vi "PRIME FITS Add Observer Info.vi"(8 "Error In":errorcluster, 10 "Observation":T2={"Priority"=0, "ID"="", "Observer"="", "Obj Name"="", "Obj Type"="", "RA and DEC String"={"RA"="HH:MM:SS.nnn", "DEC"="DEG:arcmin:arcsec.nn"}, "Filter Wheel 1"="", "Filter Wheel 2"="", "Integration Time"=0.0, "Observation Status"=enum."Error", "Offsets"={"RA"=0.0, "DEC"=0.0, "ROT"=0.0}, "Images"=0, "Dither Options"={"Dither"=enum."None", "Dither Radius"=0.0, "Dither Points"=0, "Dither Phase"=0.0}, "Comment 1"="", "Comment 2"=""}, 11 "gfits refnum":T1) -> (0 "Error Out":errorcluster, 3 "dup gfits refnum":T1)   [LabVIEW 2024, in "PRIME Detector.lvclass"]
uses:
  PRIME Detector.lvclass
  typedefs/CC cluster Observation.ctl
  Observation Queue/CC enum Observation Status.ctl
  Telescope/CC cluster Telescope Offsets.ctl
  typedefs/CC cluster Observation Dither Options.ctl
  typedefs/CC enum Dither Selection.ctl
  gfitsio/gfitsio-refnum.ctl
  gfitsio/gfitsio-write-key-string.vi
  gfitsio/gfitsio-write-key-double.vi
  gfitsio/gfitsio-write-key-integer.vi
  gfitsio/gfitsio.lvlib
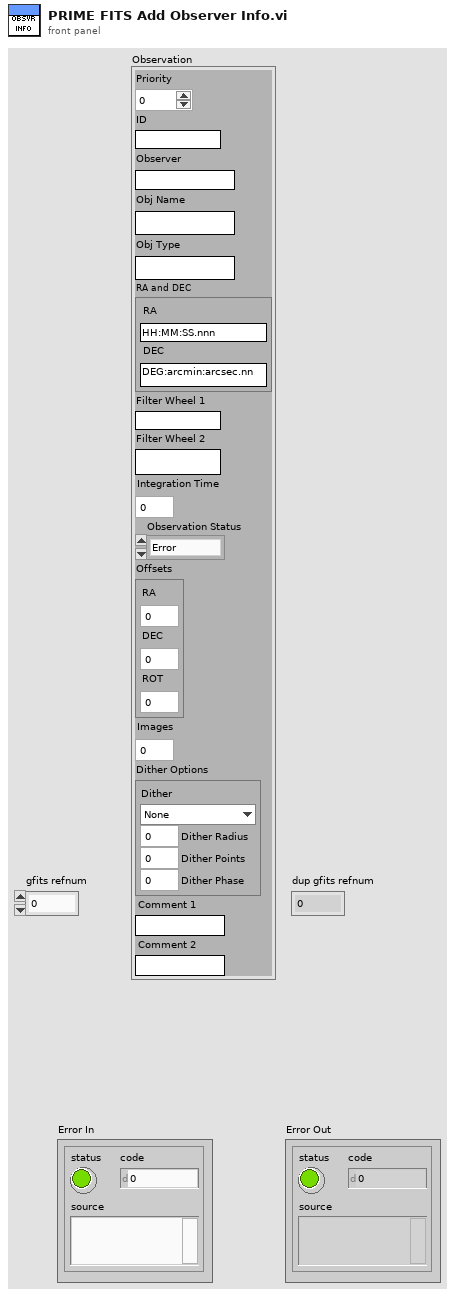
[diagram p1: front panel]
types:
  T1 = typedef "gfitsio.lvlib/gfitsio-refnum.ctl" = u64
  T2 = typedef "CC cluster Observation.ctl" = cluster{"Priority":i32, "ID":string, "Observer":string, "Obj Name":string, "Obj Type":string, "RA and DEC String":cluster{"RA":string, "DEC":string}, "Filter Wheel 1":string, "Filter Wheel 2":string, "Integration Time":dbl, "Observation Status":T3, "Offsets":T4, "Images":i32, "Dither Options":T5, "Comment 1":string, "Comment 2":string}
  T3 = typedef "CC enum Observation Status.ctl" = enum16{"Ready", "Running", "Done", "Error"}
  T4 = typedef "CC cluster Telescope Offsets.ctl" = cluster{"RA":dbl, "DEC":dbl, "ROT":dbl}
  T5 = typedef "CC cluster Observation Dither Options.ctl" = cluster{"Dither":T6, "Dither Radius":dbl, "Dither Points":i32, "Dither Phase":dbl}
  T6 = typedef "CC enum Dither Selection.ctl" = enum16{"None", "Circle", "Random"}
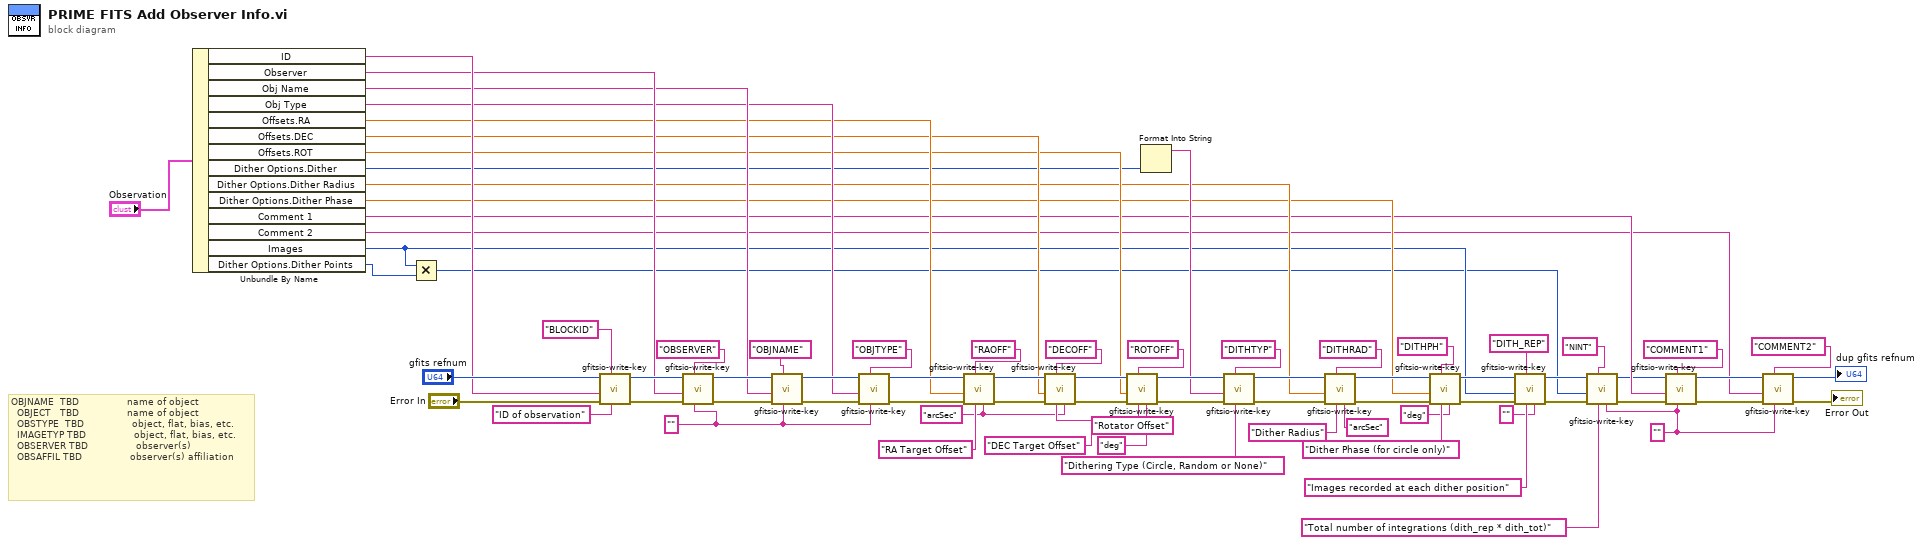
[diagram p0: block diagram]
diagram:
  w19 = "arcSec" ("units")
  w1 = "" ("comment")
  w55 = "" ("comment")
  # "OBJNAME  TBD                name of object\n  OBJECT   TBD                name of object\n  OBSTYPE  TBD                object, flat, bias, etc.\n  IMAGETYP TBD                object, flat, bias, etc.\n  OBSERVER TBD                observer(s) \n  OBSAFFIL TBD                observer(s) affiliation"
  n1 = Unbundle By Name("Observation") -> ("ID"=w65:string, "Observer"=w63:string, "Obj Name"=w61:string, "Obj Type"=w59:string, "Offsets.RA"=w57:dbl, "Offsets.DEC"=w44:dbl, "Offsets.ROT"=w41:dbl, "Dither Options.Dither"=w37:T6, "Dither Options.Dither Radius"=w32:dbl, "Dither Options.Dither Phase"=w27:dbl, "Comment 1"=w26:string, "Comment 2"=w20:string, "Images"=w7:i32, "Dither Options.Dither Points"=w6:i32)
  n2 = Multiply(x=w7, y=w6) -> (x*y=w5:i32)
  n3 = call-poly "gfitsio-write-key.vi"("comment"="ID of observation", "keyname"="BLOCKID" ("Field"), "error in (no error)"="Error In", "value"=w65, "gfits refnum"="gfits refnum") -> ("error out"=w71:errorcluster, "dup gfits refnum"=w64:T1)  [unwired: 5 in]
  n4 = call-poly "gfitsio-write-key.vi"("comment"=w55, "keyname"="OBSERVER" ("Field"), "error in (no error)"=w71, "value"=w63, "gfits refnum"=w64) -> ("error out"=w70:errorcluster, "dup gfits refnum"=w62:T1)  [unwired: 5 in]
  n5 = call-poly "gfitsio-write-key.vi"("comment"=w55, "keyname"="OBJNAME" ("Field"), "error in (no error)"=w70, "value"=w61, "gfits refnum"=w62) -> ("error out"=w69:errorcluster, "dup gfits refnum"=w60:T1)  [unwired: 5 in]
  n6 = call-poly "gfitsio-write-key.vi"("comment"=w55, "keyname"="OBJTYPE" ("Field"), "error in (no error)"=w69, "value"=w59, "gfits refnum"=w60) -> ("error out"=w68:errorcluster, "dup gfits refnum"=w58:T1)  [unwired: 5 in]
  n7 = call-poly "gfitsio-write-key.vi"("units"=w19, "comment"="RA Target Offset", "keyname"="RAOFF" ("Field"), "error in (no error)"=w68, "value"=w57, "gfits refnum"=w58) -> ("error out"=w45:errorcluster, "dup gfits refnum"=w47:T1)  [unwired: 4 in]
  n8 = call-poly "gfitsio-write-key.vi"("units"=w19, "comment"="DEC Target Offset", "keyname"="DECOFF" ("Field"), "error in (no error)"=w45, "value"=w44, "gfits refnum"=w47) -> ("error out"=w43:errorcluster, "dup gfits refnum"=w42:T1)  [unwired: 4 in]
  n9 = call-poly "gfitsio-write-key.vi"("units"="deg", "comment"="Rotator Offset", "keyname"="ROTOFF" ("Field"), "error in (no error)"=w43, "value"=w41, "gfits refnum"=w42) -> ("error out"=w39:errorcluster, "dup gfits refnum"=w38:T1)  [unwired: 4 in]
  n10 = Format Into String(w37) -> (resulting string=w36:string)  [unwired: 3 in, 1 out]
  n11 = call-poly "gfitsio-write-key.vi"("comment"="Dithering Type (Circle, Random or None)", "keyname"="DITHTYP" ("Field"), "error in (no error)"=w39, "value"=w36, "gfits refnum"=w38) -> ("error out"=w34:errorcluster, "dup gfits refnum"=w33:T1)  [unwired: 5 in]
  n12 = call-poly "gfitsio-write-key.vi"("units"="arcSec", "comment"="Dither Radius", "keyname"="DITHRAD" ("Field"), "error in (no error)"=w34, "value"=w32, "gfits refnum"=w33) -> ("error out"=w30:errorcluster, "dup gfits refnum"=w29:T1)  [unwired: 4 in]
  n13 = call-poly "gfitsio-write-key.vi"("units"="deg", "comment"="Dither Phase (for circle only)", "keyname"="DITHPH" ("Field"), "error in (no error)"=w30, "value"=w27, "gfits refnum"=w29) -> ("error out"=w15:errorcluster, "dup gfits refnum"=w14:T1)  [unwired: 4 in]
  n14 = call-poly "gfitsio-write-key.vi"("units"="", "comment"="Images recorded at each dither position", "keyname"="DITH_REP" ("Field"), "error in (no error)"=w15, "value"=w7, "gfits refnum"=w14) -> ("error out"=w13:errorcluster, "dup gfits refnum"=w12:T1)  [unwired: 4 in]
  n15 = call-poly "gfitsio-write-key.vi"("units"=w1, "comment"="Total number of integrations (dith_rep * dith_tot)", "keyname"="NINT" ("Field"), "error in (no error)"=w13, "value"=w5, "gfits refnum"=w12) -> ("error out"=w10:errorcluster, "dup gfits refnum"=w11:T1)  [unwired: 4 in]
  n16 = call-poly "gfitsio-write-key.vi"("comment"=w1, "keyname"="COMMENT1" ("Field"), "error in (no error)"=w10, "value"=w26, "gfits refnum"=w11) -> ("error out"=w24:errorcluster, "dup gfits refnum"=w25:T1)  [unwired: 5 in]
  n17 = call-poly "gfitsio-write-key.vi"("comment"=w1, "keyname"="COMMENT2" ("Field"), "error in (no error)"=w24, "value"=w20, "gfits refnum"=w25) -> ("error out"=→"Error Out":errorcluster, "dup gfits refnum"=→"dup gfits refnum":T1)  [unwired: 5 in]
